vi "LuaVIEW Get Task Script Directory.vi"(5 "LuaVIEW reference in":T1, 11 "error in (no error)":errorcluster) -> (4 "task script directory":path, 6 "LuaVIEW reference out":T1, 15 "error out":errorcluster)   [LabVIEW 2012]
doc: "Returns the directory holding the task script. When not a task, task script remote, or task script provided as a string, an empty path and error is returned."
uses:
  typedefs/t_LuaVIEW Reference.ctl
  typedefs/t_LuaVIEW Task State Methods.ctl
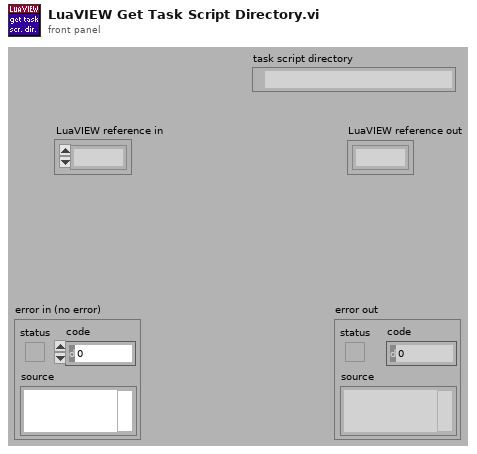
[diagram p1: front panel]
types:
  T1 = typedef "t_LuaVIEW Reference.ctl" = refnum<k1>
  T2 = typedef "t_LuaVIEW Task State Methods.ctl" = enum16{"cleanup", "set initial", "set mode", "set active mode", "set error", "get task info", "get script info", "set signal", "clear signal", "test handled", "test delegated", "test signal", "handle signal", "delegate signal", "allow signal", "disallow signal", "disallow all", "signals?", "delegated signals?", "protection++", "protection--", "protection=0", "message", "next message", "pop message", "message available?", "force stop", "set swap preps", "apply swap preps"}
  T3 = typedef "t_LuaVIEW Task State Pane.ctl" = refnum<vi>
  T4 = typedef "LuaVIEW Task Info.ctl" = cluster{"main script":string, "identifier":string, "class":string, "description":string, "mode":T5, "handler":string, "LuaVIEW reference":T1, "scripts":i32, "hide":bool, "active":bool, "error msg":string, "defer":bool, "launch":enum16{"asynchronous", "manual", "synchronous"}, "main path valid":bool, "start time":dbl, "swap time":dbl, "task VI":refnum<vi>, "prefsys":enum32{"invalid execution system", "user interface", "standard", "instrument i/o", "data acquisition", "other 1", "other 2", "same as caller"}, "priority":enum32{"invalid priority", "background priority", "normal priority", "above normal priority", "high priority", "time critical priority", "subroutine"}, "signal flags":u32, "allow mask":u32, "handle mask":u32, "disallow manual":bool}
  T5 = typedef "t_LuaVIEW Task Modes.ctl" = enum16{"initializing", "running", "executing", "paused", "error", "swapping"}
  T6 = typedef "LuaVIEW Script Info.ctl" = cluster{"path":path, "description":string, "text":string, "parent index":i32, "version":string}
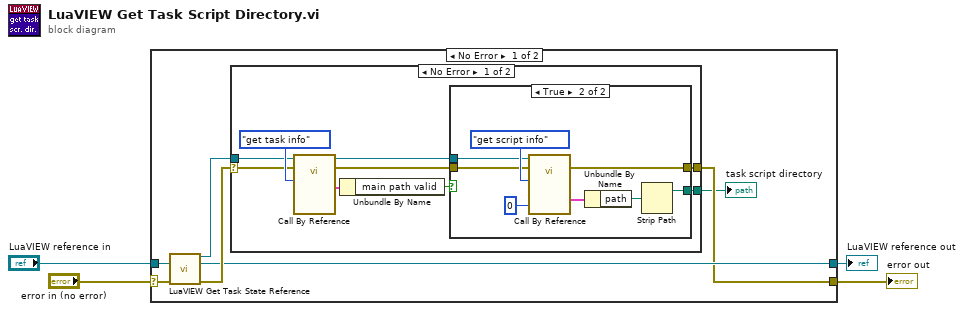
[diagram p0: block diagram]
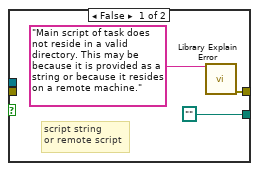
[diagram p2: hidden frame]
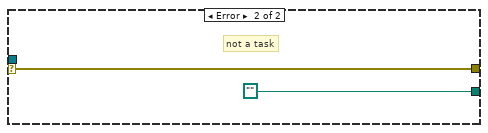
[diagram p3: hidden frame]
diagram:
  n1 = case shown="No Error" "error in (no error)" {
    selector: "error in (no error)" -> [w11 w35]
    tunnel: [w7 w34] -> w4
    tunnel: [w6 w35] -> w3
    tunnel: "LuaVIEW reference in" -> [w10 w34]
    frame No Error {
      n2 = call "LuaVIEW Get Task State Reference.vi"("LuaVIEW reference in"=w10, "error in (no error)"=w11) -> ("task state reference"=w8:T3, "LuaVIEW reference out"=w7:T1, "error out"=w9:errorcluster)  [unwired: 11 in]
      n3 = case shown="No Error" w9 {
        selector: w9 -> [w17 w32]
        tunnel: w8 -> [w18 _]
        tunnel: [w20 path ""] -> w5
        tunnel: [w12 w32] -> w6
        frame No Error {
          n4 = call-by-ref "?"(reference=w18, error in=w17, "method"=t_LuaVIEW_Task_State_Methods."get task info") -> (reference out=w14:T3, error out=w13:errorcluster, "task info {get task info}"=w16:T4)  [unwired: 10 in, 4 out]
          n5 = Unbundle By Name(w16) -> ("main path valid"=w15:bool)
          n6 = case shown="True" w15 {
            tunnel: [path "" w27] -> w20
            tunnel: w14 -> [_ w26]
            tunnel: w13 -> [_ w25]
            tunnel: [w21 w24] -> w12
            frame False {
              # "script string\nor remote script"
              n7 = call "Library Explain Error.vi"("explanation prefix (none)"="Main script of task does not reside in a valid directory. This may be because it is provided as a string or because it resides on a remote machine." ("string out")) -> ("explained error"=w21:errorcluster)  [unwired: 14 in]
            }
            frame True {
              n8 = call-by-ref "?"(reference=w26, error in=w25, "method"=t_LuaVIEW_Task_State_Methods."get script info", "script index"=0) -> (error out=w24:errorcluster, "script info"=w31:T6)  [unwired: 9 in, 5 out]
              n9 = Unbundle By Name(w31) -> ("path"=w28:path)
              n10 = Strip Path(path=w28) -> (stripped path=w27:path)  [unwired: 1 out]
            }
          }
        }
        frame Error {
          # "not a task"
        }
      }
      "task script directory" <- w5
    }
    frame Error {
    }
  }
  "LuaVIEW reference out" <- w4
  "error out" <- w3
